vi "hdf5 image file ref FGV.vi"(8 "error in (no error)":errorcluster, 9 "module path in":path, 10 "command":enum16{"set", "get"}(ring)=enum."get", 11 "Python session":refnum<k35>) -> (0 "error out":errorcluster, 1 "module path":path, 3 "Python session":refnum<k35>)   [LabVIEW 2020]
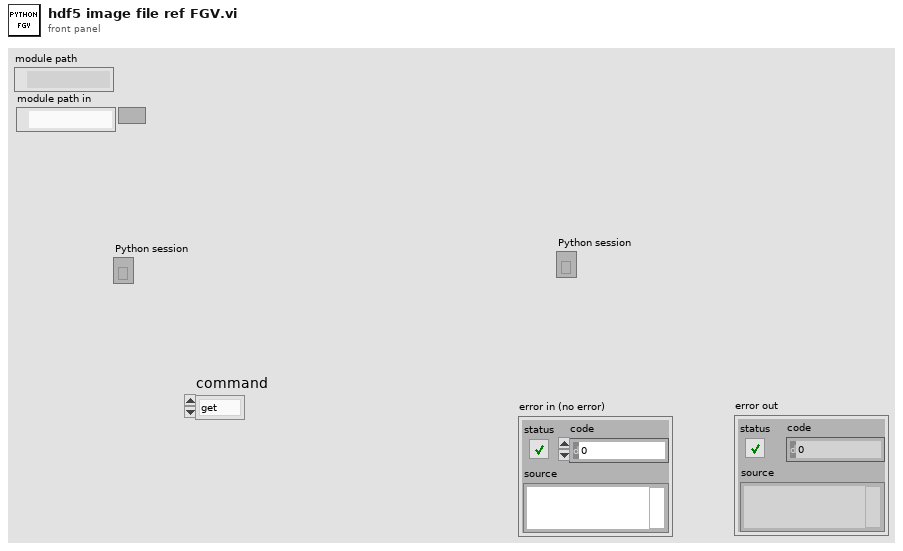
[diagram p1: front panel]
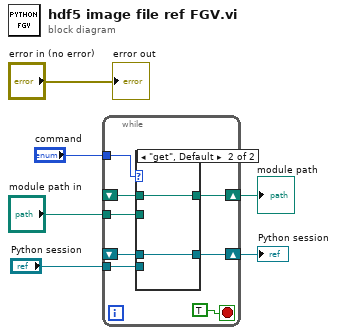
[diagram p0: block diagram]
diagram:
  n1 = while {
    shift-right: [w11] -> w3
    shift-left: _ -> [w12]
    tunnel: "command" -> [w13]
    tunnel: "Python session" -> [w10]
    tunnel: "module path in" -> [w8]
    shift-right: [w9] -> w1
    shift-left: _ -> [w7]
    stop <- TRUE stop-if-true
    n2 = case shown="\"get\", Default" w13 {
      tunnel: w12 -> [_ w18]
      tunnel: [w16 w18] -> w11
      tunnel: w10 -> [w16 _]
      tunnel: [w15 w17] -> w9
      tunnel: w8 -> [w15 _]
      tunnel: w7 -> [_ w17]
      frame "set" {
      }
      frame "get", Default {
      }
    }
  }
  "Python session" <- w3
  "module path" <- w1
  "error out" <- "error in (no error)"
